vi "dfd_NStage MRate Quantization.vi"(5 "scale by Power of 2?":bool, 6 "gain wl":i16=16, 7 "scale type":T1=enum."Time Domain 1-Norm", 8 "error in (no error)":errorcluster, 9 "last FIR idx":i32, 10 "coef wl":i16[](array[numeric]), 11 "multirate filters in":T2[](array[typedef]) {"mMRate_SumWl" min=1 max=32 step=1; "mMRate_InputIwl" min=1 max=32 step=1; "mMRate_GainWl" min=1 max=32 step=1; "mMRate_OutputWl" min=1 max=32 step=1; "mMRate_InputWl" min=1 max=32 step=1; "mMRate_CoefWl" min=1 max=32 step=1; "mMRate_Mode" items=["Default"=-1, "No Rate Change"=0, "Interpolation"=1, "Decimation"=2, "Interpolated"=3, "Rational"=4]}) -> (0 "error out":errorcluster, 2 "scaled gain":dbl, 3 "multirate filters out":T2[](array[typedef]) {"mMRate_SumWl" min=1 max=32 step=1; "mMRate_InputIwl" min=1 max=32 step=1; "mMRate_GainWl" min=1 max=32 step=1; "mMRate_OutputWl" min=1 max=32 step=1; "mMRate_InputWl" min=1 max=32 step=1; "mMRate_CoefWl" min=1 max=32 step=1; "mMRate_Mode" items=["Default"=-1, "No Rate Change"=0, "Interpolation"=1, "Decimation"=2, "Interpolated"=3, "Rational"=4]})   [LabVIEW 2017, in "NI_DigFilter_FXP.lvlib"]
uses:
  <vilib>/addons/Digital Filter Design/NI_DigFilter_FXP.lvlib
  <vilib>/addons/Digital Filter Design/_Objects.llb/DFD Multirate Filter Obj.ctl
  <vilib>/addons/Digital Filter Design/_Objects.llb/DFD Multirate Mode.ctl
  <vilib>/addons/Digital Filter Design/_Objects.llb/DFD Coef Norm Type.ctl
  <vilib>/addons/Digital Filter Design/_Objects.llb/DFD Round-off Mode.ctl
  <vilib>/addons/Digital Filter Design/_Objects.llb/DFD FXP MRate Multiply Mode.ctl
  <vilib>/addons/Digital Filter Design/_Objects.llb/DFD FXP MRate Internal Precision Mode.ctl
  <vilib>/addons/Digital Filter Design/NI_DigFilterLicensed.lvlib
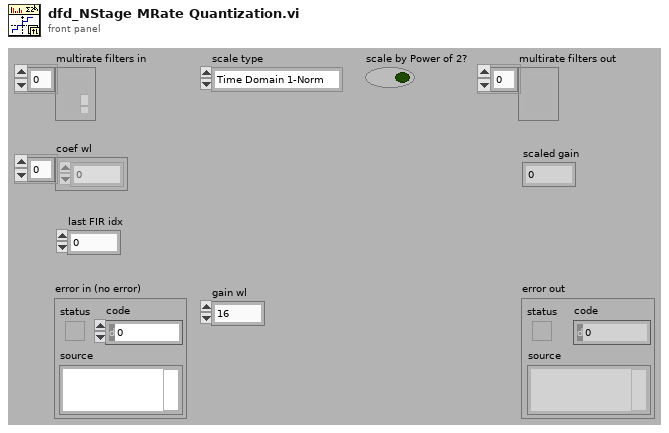
[diagram p1: front panel]
types:
  T1 = typedef "NI_DigFilterLicensed.lvlib/DFD Coef Norm Type.ctl" = enum16{"No Norm", "Time Domain 1-Norm", "Time Domain 2-Norm", "Time Domain Inf-Norm"}
  T2 = typedef "NI_DigFilterLicensed.lvlib/DFD Multirate Filter Obj.ctl" = cluster{"mMRate_Structure":enum16{"CIC", "FIR", "IIR", "Lattice"}, "mMRate_Mode":T3, "mMRate_Factor":i32, "mMRate_FIRParams":cluster{"mMRate_FIR_H":dbl[], "mMRate_FIR_IsNyquist?":bool, "mMRate_FIR_IsSymmetric?":bool}, "mMRate_CICParams":cluster{"mMRate_CIC_#Stage":i32, "mMRate_CIC_Lag":i32, "mMRate_CIC_Type":enum16{"Lowpass", "Highpass"}}, "mMRate_Order":i32, "mMRate_Version":string, "mMRate_Comments":string, "mMRate_RationalFactor":cluster{"mMRate_L":i32, "mMRate_M":i32}, "mMRate_Fs":dbl, "mMRate_Quantized?":bool, "mMRate_QFilterGain":dbl, "mMRate_CoefWl":i16, "mMRate_Scaling":cluster{"mMRate_ScaleByPowerOf2?":bool, "mMRate_ScaleType":T1}, "mMRate_InputWl":i16, "mMRate_OutputWl":i16, "mMRate_OutputMode":T4, "mMRate_MultMode":T5, "mMRate_BitPruning":bool, "mMRate_GainWl":i16, "mMRate_OutputFwl":i16, "mMRate_SumIwl":i16, "mMRate_InputIwl ":i16, "mMRate_SumWl":i16, "mMRate_CoefIwl":i16}
  T3 = typedef "NI_DigFilterLicensed.lvlib/DFD Multirate Mode.ctl" = i16
  T4 = typedef "NI_DigFilterLicensed.lvlib/DFD Round-off Mode.ctl" = enum16{"Nearest", "Truncation"}
  T5 = typedef "NI_DigFilterLicensed.lvlib/DFD FXP MRate Multiply Mode.ctl" = enum16{"Truncated", "Full"}
  T6 = typedef "NI_DigFilterLicensed.lvlib/DFD FXP MRate Internal Precision Mode.ctl" = enum16{"Truncated", "Full"}
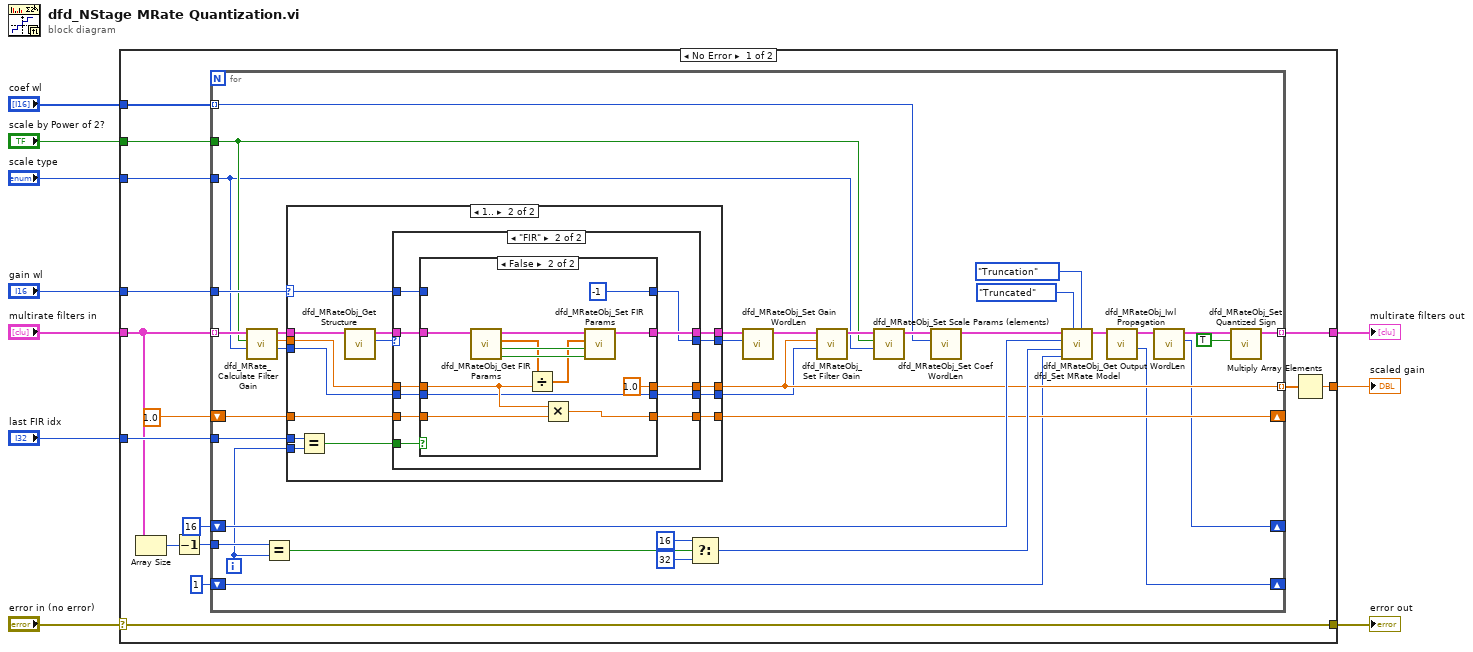
[diagram p0: block diagram]
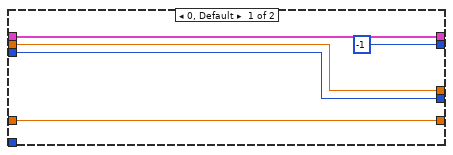
[diagram p2: hidden frame]
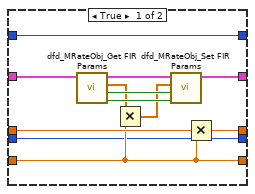
[diagram p4: hidden frame]
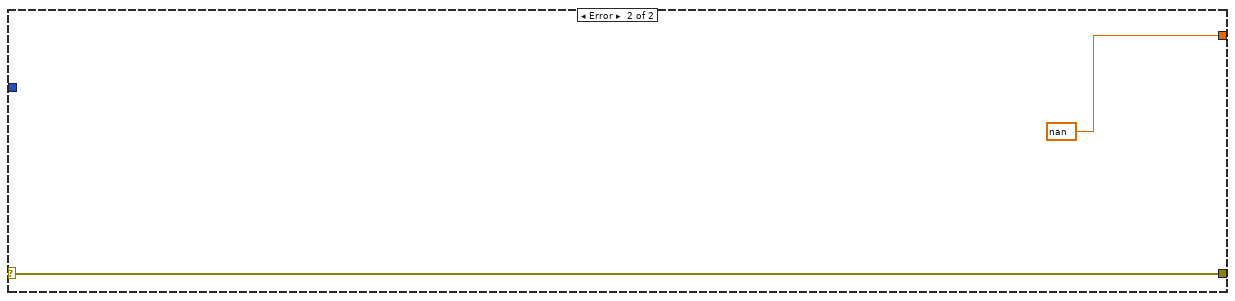
[diagram p5: hidden frame]
diagram:
  n1 = case shown="No Error" "error in (no error)" {
    selector: "error in (no error)" -> [w22 w123]
    tunnel: "multirate filters in" -> [w17 _]
    tunnel: "scale type" -> [w25 _]
    tunnel: "coef wl" -> [w21 _]
    tunnel: [w24 _] -> w8
    tunnel: "scale by Power of 2?" -> [w23 _]
    tunnel: [w14 nan ("filter gain")] -> w7
    tunnel: [w22 w123] -> w4
    tunnel: "gain wl" -> [w19 _]
    tunnel: "last FIR idx" -> [w20 _]
    frame No Error {
      n2 = Array Size(array=w17) -> (size(s)=w16:i32)
      n3 = Decrement(x=w16) -> (x-1=w11:i32)
      n4 = for {
        tunnel: w25 -> [w35]
        tunnel: [w59] -> w24 mode=indexing
        tunnel: w23 -> [w36]
        tunnel: [w34] -> w15 mode=indexing
        tunnel: w17 -> [w41] mode=indexing
        tunnel: w21 -> [w44] mode=indexing
        tunnel: w20 -> [w48]
        tunnel: w19 -> [w50]
        shift-right: [w32] -> _
        shift-left: i16 16 ("input wl") -> [w54]
        tunnel: w11 -> [w56]
        shift-right: [w45] -> _
        shift-left: 1.0 -> [w46]
        shift-right: [w29] -> _
        shift-left: i16 1 -> [w30]
        i -> [w47]
        n5 = call <vilib>:"dfd_MRate_Calculate Filter Gain.vi"("scale type"=w35, "scale by Power of 2?"=w36, "multirate filter in"=w41) -> ("sum iwl"=w38:i16, "scaled gain"=w39:dbl, "dup multirate filter"=w40:T2)  [unwired: 6 out]
        n6 = Equal?(x=w56, y=w47) -> (x = y?=w55:bool)
        n7 = case shown="1.." w50 {
          selector: w50 -> [_ w71]
          tunnel: w40 -> [w64 w81]
          tunnel: [w64 w79] -> w37
          tunnel: [i16 -1 ("gain wl") w78] -> w49
          tunnel: w48 -> [_ w77]
          tunnel: w47 -> [_ w76]
          tunnel: w46 -> [w66 w74]
          tunnel: [w66 w72] -> w45
          tunnel: w39 -> [w63 w70]
          tunnel: w38 -> [w62 w68]
          tunnel: [w63 w69] -> w34
          tunnel: [w62 w67] -> w33
          frame 0, Default {
          }
          frame 1.. {
            n8 = Equal?(x=w77, y=w76) -> (x = y?=w73:bool)
            n9 = call <vilib>:"dfd_MRateObj_Get Structure.vi"("multirate filter in"=w81) -> ("structure"=w75:enum16{"CIC", "FIR", "IIR", "Lattice"}, "dup multirate filter"=w80:T2)  [unwired: 9 out]
            n10 = case shown="\"FIR\"" w75 {
              tunnel: w80 -> [w86 w91]
              tunnel: [w86 w97] -> w79
              tunnel: [w82 w94] -> w78
              tunnel: w74 -> [w85 w93]
              tunnel: w73 -> [_ w96]
              tunnel: [w85 w92] -> w72
              tunnel: w71 -> [w82 w95]
              tunnel: [w84 w87] -> w69
              tunnel: w70 -> [w84 w90]
              tunnel: w68 -> [w83 w89]
              tunnel: [w83 w88] -> w67
              frame "CIC", Default {
              }
              frame "FIR" {
                n11 = case shown="False" w96 {
                  tunnel: [w109 w122] -> w97
                  tunnel: w91 -> [w108 w113]
                  tunnel: w95 -> [w104 _]
                  tunnel: [w104 i16 -1 ("gain wl")] -> w94
                  tunnel: w93 -> [w100 w115]
                  tunnel: [w100 w114] -> w92
                  tunnel: w90 -> [w101 w112]
                  tunnel: w89 -> [w98 w111]
                  tunnel: [w98 w111] -> w88
                  tunnel: [w99 1.0] -> w87
                  frame True {
                    n12 = call <vilib>:"dfd_MRateObj_Get FIR Params.vi"("multirate filter in"=w108) -> ("is symmetric?"=w105:bool, "is Nyquist?"=w106:bool, "h(n)"=w103:dbl[], "dup multirate filter"=w107:T2)  [unwired: 7 out]
                    n13 = Multiply(x=w103, y=w100) -> (x*y=w102:dbl[])
                    n14 = call <vilib>:"dfd_MRateObj_Set FIR Params.vi"("is symmetric?"=w105, "is Nyquist?"=w106, "h(n)"=w102, "multirate filter in"=w107) -> ("multirate filter out"=w109:T2)  [unwired: 7 out]
                    n15 = Multiply(x=w101, y=w100) -> (x*y=w99:dbl)
                  }
                  frame False {
                    n16 = call <vilib>:"dfd_MRateObj_Get FIR Params.vi"("multirate filter in"=w113) -> ("is symmetric?"=w119:bool, "is Nyquist?"=w120:bool, "h(n)"=w118:dbl[], "dup multirate filter"=w121:T2)  [unwired: 7 out]
                    n17 = Divide(x=w118, y=w112) -> (x/y=w117:dbl[])
                    n18 = Multiply(x=w112, y=w115) -> (x*y=w114:dbl)
                    n19 = call <vilib>:"dfd_MRateObj_Set FIR Params.vi"("is symmetric?"=w119, "is Nyquist?"=w120, "h(n)"=w117, "multirate filter in"=w121) -> ("multirate filter out"=w122:T2)  [unwired: 7 out]
                  }
                }
              }
            }
          }
        }
        n20 = Select(t=i16 16, s=w55, f=i16 32) -> (s? t:f=w51:i16)
        n21 = call <vilib>:"dfd_MRateObj_Set Gain WordLen.vi"("gain wl"=w49, "multirate filter in"=w37) -> ("multirate filter out"=w42:T2)  [unwired: 9 out]
        n22 = call <vilib>:"dfd_MRateObj_Set Filter Gain.vi"("sum iwl"=w33, "gain"=w34, "multirate filter in"=w42) -> ("multirate filter out"=w43:T2)  [unwired: 8 out]
        n23 = call <vilib>:"dfd_MRateObj_Set Scale Params (elements).vi"("scale type"=w35, "scale by Power of 2?"=w36, "multirate filter in"=w43) -> ("multirate filter out"=w61:T2)  [unwired: 8 out]
        n24 = call <vilib>:"dfd_MRateObj_Set Coef WordLen.vi"("coef wl"=w44, "multirate filter in"=w61) -> ("multirate filter out"=w31:T2)  [unwired: 9 out]
        n25 = call <vilib>:"dfd_Set MRate Model.vi"("output rounding mode"=DFD_Round-off_Mode."Truncation" ("output round-off mode"), "internal precision"=DFD_FXP_MRate_Internal_Precision_Mode."Truncated", "input iwl"=w30, "output wl"=w51, "input wl"=w54, "multirate filter in"=w31) -> ("multirate filter out"=w28:T2)  [unwired: 1 in, 4 out]
        n26 = call <vilib>:"dfd_MRateObj_Iwl Propagation.vi"("multirate filter"=w28) -> ("Actual Output iwl"=w29:i16, "dup multirate filter"=w27:T2)  [unwired: 9 out]
        n27 = call <vilib>:"dfd_MRateObj_Get Output WordLen.vi"("multirate filter in"=w27) -> ("output wl"=w32:i16, "dup multirate filter"=w26:T2)  [unwired: 9 out]
        n28 = call <vilib>:"dfd_MRateObj_Set Quantized Sign.vi"("Quantized?"=TRUE, "multirate filter in"=w26) -> ("multirate filter out"=w59:T2)  [unwired: 9 out]
      }
      n29 = Multiply Array Elements(1:w15) -> (0:w14:dbl)
    }
    frame Error {
    }
  }
  "multirate filters out" <- w8
  "error out" <- w4
  "scaled gain" <- w7
